vi "Set Baud Rate.vi"(8 "error in (no error)":errorcluster, 10 "baud rate":u8(ring) items=["9600", "38400", "19200"], 11 "RRG in":refnum<class "Eltochpribor RRG.lvclass">) -> (0 "error out":errorcluster, 3 "RRG out":refnum<class "Eltochpribor RRG.lvclass">)   [LabVIEW 2015, in "Eltochpribor RRG.lvclass"]
doc: "Sets communication baud rate."
uses:
  Eltochpribor RRG.lvclass
  Modbus Client/PL Modbus Client.lvclass
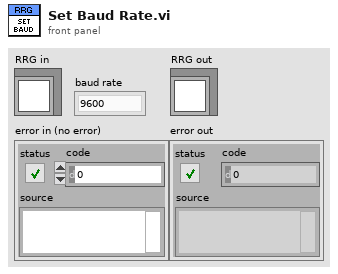
[diagram p1: front panel]
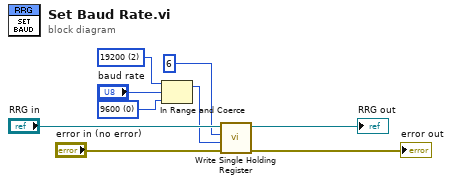
[diagram p0: block diagram]
diagram:
  w2 = u8 0 items=["9600", "38400", "19200"] ("baud rate")
  w3 = u8 2 items=["9600", "38400", "19200"] ("baud rate")
  n1 = In Range and Coerce(upper limit=w3, x="baud rate", lower limit=w2) -> (coerced(x)=w1:u8)  [unwired: 1 out]
  n2 = call "Write Single Holding Register.vi"("error in (no error)"="error in (no error)", "value"=w1, "address"=u16 6, "MODBUS in"="RRG in") -> ("error out"=→"error out":errorcluster, "MODBUS out"=→"RRG out":refnum<class "Eltochpribor RRG.lvclass">)  [unwired: 6 in]
